vi "Coupling.vi"(0 "VISA IN":refnum<visa-resource-name>, 1 "Sweep Mode(ALL or NONE)":string(combo)="ALL", 2 "Parameters to Couple":T1(ring), 3 "Measurement Name":string, 4 "Time Domain Trace Coupling ON/OFF":bool=TRUE, 5 "error in":errorcluster, 7 "Channel":i32=1) -> (14 "VISA Out":refnum<visa-resource-name>, 19 "error out":errorcluster)   [LabVIEW 2018, in "PNA-X.lvlib"]
uses:
  PNA-X.lvlib
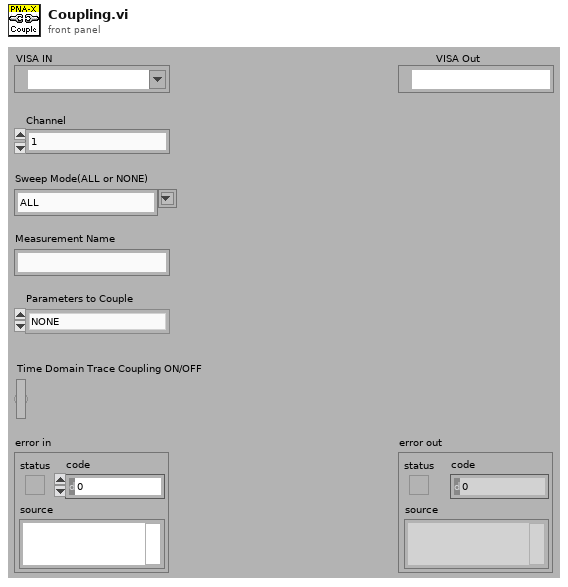
[diagram p1: front panel]
types:
  T1 = enum16{"NONE", "Stimulus", "State (ON/OFF)", "Stimulus, State", "Window (Kaiser Bets / Impulse Width)", "Window, Stimulus", "Window, State", "Window, State, Stimulus", "Mode (Low Pass Impulse, Low Pass Step, Band Pass)", "Mode, Stimulus", "Mode, State", "Mode, State, Stimulus", "Mode, Window", "Mode, Window, Stimulus", "Mode, Window, State", "Mode, Window, State, Stimulus", "Distance Marker Units", "Distance, Stimulus", "Distance, State", "Distance, State, Stimulus", "Distance, Window", "Distance, Window, Stimulus", "Distance, Window, State", "Distance, Window, State, Stimulus", "Distance, Mode", "Distance, Mode, Stimulus", "Distance, Mode, State", "Distance, Mode, State, Stimulus", "Distance, Mode, Window", "Distance, Mode, Window, Stimulus", "Distance, Mode, Window, State", "Distance, Mode, Window, State, Stimulus"}
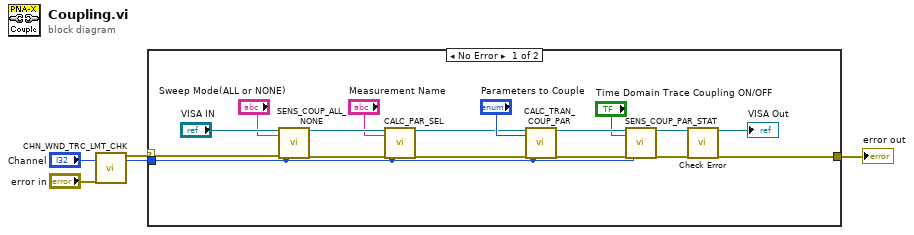
[diagram p0: block diagram]
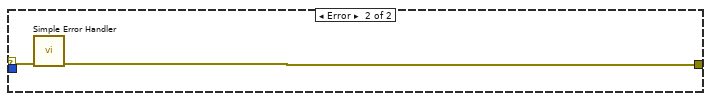
[diagram p2: hidden frame]
diagram:
  n1 = call "CHN_WND_TRC_LMT_CHK.vi"("Channel"="Channel", "error in"="error in") -> ("error out"=w2:errorcluster, "Channel"=w1:i32)  [unwired: 13 in, 3 out]
  n2 = case shown="No Error" w2 {
    selector: w2 -> [w18 w24]
    tunnel: [w22 w23] -> w4
    tunnel: w1 -> [w7 _]
    frame No Error {
      n3 = call "SENS_COUP_ALL_NONE.vi"("VISA IN"="VISA IN", "Sweep Mode(ALL or NONE)"="Sweep Mode(ALL or NONE)", "error in"=w18, "Channel"=w7) -> ("VISA Out"=w11:refnum<visa-resource-name>, "error out"=w9:errorcluster)  [unwired: 14 in]
      n4 = call "CALC_PAR_SEL.vi"("VISA IN"=w11, "Measurement"="Measurement Name", "error in"=w9, "Channel"=w7) -> ("VISA Out"=w10:refnum<visa-resource-name>, "error out"=w8:errorcluster)  [unwired: 14 in]
      n5 = call "CALC_TRAN_COUP_PAR.vi"("VISA IN"=w10, "Parameters to Couple"="Parameters to Couple", "error in"=w8, "Channel"=w7) -> ("VISA Out"=w17:refnum<visa-resource-name>, "error out"=w19:errorcluster)  [unwired: 14 in]
      n6 = call "SENS_COUP_PAR_STAT.vi"("VISA IN"=w17, "Time Domain Trace Coupling ON/OFF"="Time Domain Trace Coupling ON/OFF", "error in"=w19, "Channel"=w7) -> ("VISA Out"=w16:refnum<visa-resource-name>, "error out"=w20:errorcluster)  [unwired: 14 in]
      n7 = call "Check Error.vi"("VISA Resource Name"=w16, "error in (no error)"=w20) -> ("dup VISA session"=→"VISA Out":refnum<visa-resource-name>, "error out"=w22:errorcluster)  [unwired: 16 in]
    }
    frame Error {
      n8 = call <vilib>:"Simple Error Handler.vi"("error in (no error)"=w24) -> ("error out"=w23:errorcluster)  [unwired: 4 in, 4 out]
    }
  }
  "error out" <- w4
